vi "IQ_Add_CP.vi"(11 "IQ":cdb[](array[numeric])) -> (3 "IQ_CP":cdb[](array[numeric]))   [LabVIEW 2015]
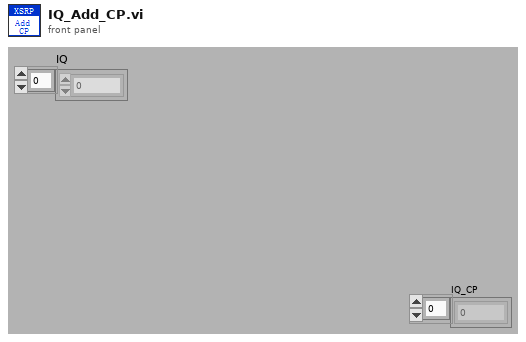
[diagram p1: front panel]
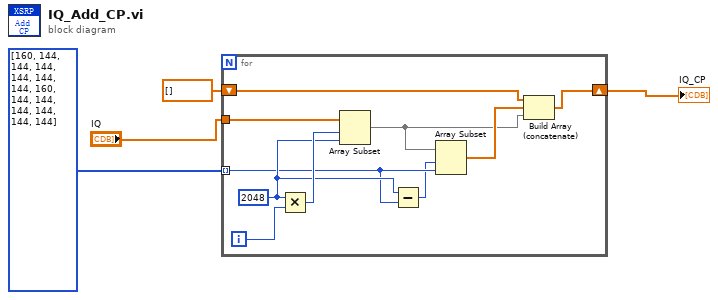
[diagram p0: block diagram]
diagram:
  n1 = for {
    tunnel: "IQ" -> [w14]
    shift-right: [w6] -> w3
    shift-left: cdb[] [] -> [w5]
    tunnel: i32[] [160, 144, 144, 144, 144, 144, 144, 160, 144, 144, 144, 144, 144, 144] -> [w10] mode=indexing
    i -> [w13]
    w11 = 2048 ("x")
    n2 = Multiply(x=w11, y=w13) -> (x*y=w12:i32)
    n3 = Array Subset(array=w14, index=w12, length=w11) -> (w7:cdb[])
    n4 = Subtract(x=w11, y=w10) -> (x-y=w9:i32)
    n5 = Array Subset(array=w7, index=w9, length=w10) -> (w8:cdb[])
    n6 = Build Array (concatenate)(w5, w8, w7) -> (w6:cdb[])
  }
  "IQ_CP" <- w3
